vi "Post_Build_Move_Runtime.vi"(8 "error in (no error)":errorcluster, 9 "Files in":path[](array[path])) -> (0 "error out":errorcluster, 1 "Files out":path[](array[path]), 2 "Path":path, 3 "Runtime Path":path, 5 "LV Version":string)   [LabVIEW 2022 SP3]
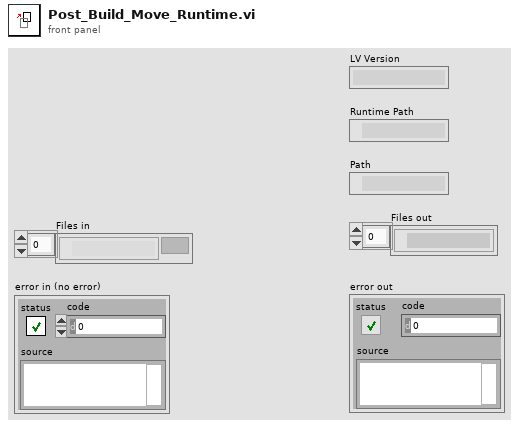
[diagram p1: front panel]
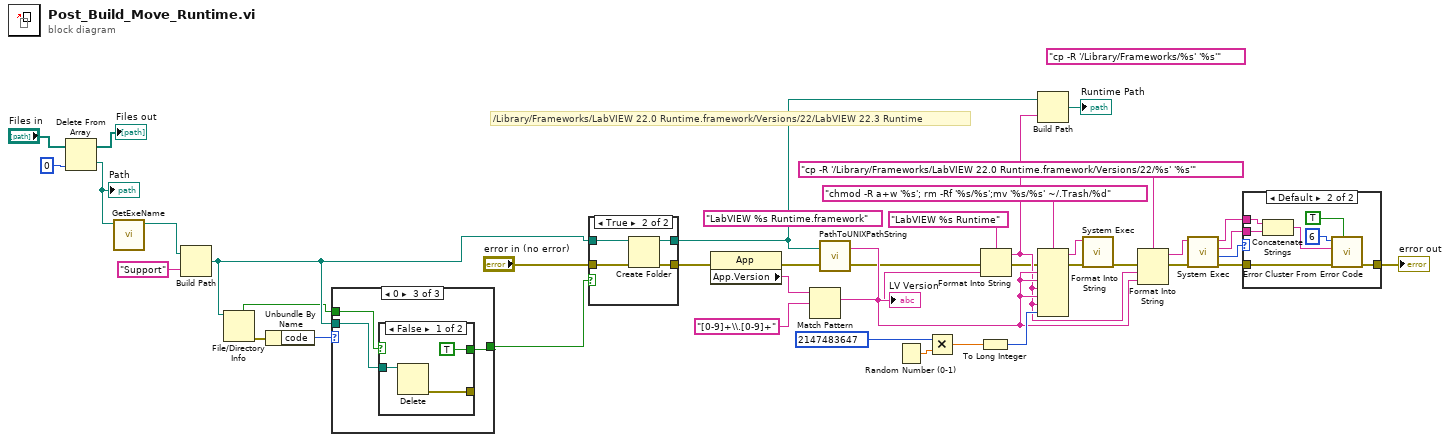
[diagram p0: block diagram]
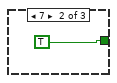
[diagram p5: hidden frame]
diagram:
  (unwired) "LabVIEW %s Runtime.framework" ("UNIX Path")
  (unwired) "cp -R '/Library/Frameworks/%s' '%s'" ("UNIX Path")
  # "/Library/Frameworks/LabVIEW 22.0 Runtime.framework/Versions/22/LabVIEW 22.3 Runtime"
  n1 = Delete From Array(array="Files in", index=0) -> (deleted portion=w2:path, array with subset deleted=→"Files out":path[])  [unwired: 1 in]
  "Path" <- w2
  n2 = call "GetExeName.vi"("Path"=w2) -> ("new path"=w1:path)  [unwired: 10 in]
  n3 = Build Path(base path=w1, name or relative path="Support") -> (appended path=w10:path)
  n4 = File/Directory Info(path=w10) -> (directory=w7:bool, error out=w5:errorcluster)  [unwired: 1 in, 5 out]
  n5 = Unbundle By Name(w5) -> ("code"=w6:i32)
  n6 = case shown="0" w6 {
    tunnel: w7 -> [_ _ w44]
    tunnel: w10 -> [_ _ w43]
    tunnel: [_ TRUE w42] -> w9
    frame Default {
    }
    frame 7 {
    }
    frame 0 {
      n7 = case shown="False" w44 {
        tunnel: w43 -> [w47 _]
        tunnel: [w46 _] -> _
        tunnel: [TRUE _] -> w42
        frame False {
          n8 = Delete(path (use dialog)=w47) -> (error out=w46:errorcluster)  [unwired: 4 in, 2 out]
        }
        frame True {
        }
      }
    }
  }
  n9 = case shown="True" w9 {
    tunnel: w10 -> [w48 w53]
    tunnel: "error in (no error)" -> [w49 w52]
    tunnel: [w49 w51] -> w17
    tunnel: [w48 w50] -> w29
    frame False {
    }
    frame True {
      n10 = Create Folder(path (use dialog)=w53, error in=w52) -> (created path=w50:path, error out=w51:errorcluster)  [unwired: 1 in, 1 out]
    }
  }
  n11 = property class="App"(error in=w17) -> (error out=w18:errorcluster, "App.Version"=w11:string)  [unwired: 1 in, 1 out]
  n12 = Match Pattern(string=w11, regular expression="[0-9]+\\.[0-9]+") -> (match substring=w25:string)  [unwired: 1 in, 3 out]
  n13 = call <vilib>:"PathToUNIXPathString.vi"("error in (no error)"=w18, "LV Path"=w29) -> ("error out"=w27:errorcluster, "UNIX Path"=w37:string)
  "LV Version" <- w37
  n14 = Random Number (0-1)() -> (number: 0 to 1=w35:dbl)
  n15 = Multiply(x=2147483647, y=w35) -> (x*y=w36:dbl)
  n16 = To Long Integer(number=w36) -> (32bit integer=w38:i32)
  n17 = Format Into String(format string="LabVIEW %s Runtime" ("UNIX Path"), error in=w27, w25) -> (resulting string=w33:string, error out=w26:errorcluster)  [unwired: 1 in]
  n18 = Build Path(base path=w29, name or relative path=w33) -> (appended path=→"Runtime Path":path)
  n19 = Format Into String(format string="chmod -R a+w '%s'; rm -Rf '%s/%s';mv '%s/%s' ~/.Trash/%d" ("UNIX Path"), error in=w26, w37, w37, w33, w37, w33, w38) -> (resulting string=w21:string, error out=w22:errorcluster)  [unwired: 1 in]
  n20 = call <vilib>:"System Exec.vi"("error in (no error)"=w22, "command line"=w21) -> ("error out"=w28:errorcluster)  [unwired: 6 in, 3 out]
  n21 = Format Into String(format string="cp -R '/Library/Frameworks/LabVIEW 22.0 Runtime.framework/Versions/22/%s' '%s'" ("UNIX Path"), error in=w28, w33, w37) -> (resulting string=w14:string, error out=w13:errorcluster)  [unwired: 1 in]
  n22 = call <vilib>:"System Exec.vi"("error in (no error)"=w13, "command line"=w14) -> ("error out"=w16:errorcluster, "return code"=w15:i32, "standard error"=w20:string, "standard output"=w19:string)  [unwired: 6 in]
  n23 = case shown="Default" w15 {
    tunnel: [w54 w56] -> w32
    tunnel: w16 -> [w54 w57]
    tunnel: w19 -> [_ w60]
    tunnel: w20 -> [_ w59]
    frame 0 {
    }
    frame Default {
      n24 = Concatenate Strings(w60, w59) -> (w58:string)
      n25 = call <vilib>:"Error Cluster From Error Code.vi"("show call chain? (False)"=TRUE, "error in (no error)"=w57, "error message (\"\")"=w58, "error code (0)"=6) -> ("error out"=w56:errorcluster)  [unwired: 5 in]
    }
  }
  "error out" <- w32
